vi "CRYNot.ch Resonance.vi"(8 "Y ref":dbl=1.0, 9 "Curve in":cluster{"x":dbl, "y":dbl, "z":dbl}[](array[cluster]) {"z" format="%.2f"; "y" format="%.2f"; "x" format="%.2f"}, 10 "Fraction down (1/sqrt(2))":dbl=0.2928932188134525 format="%.4f", 11 "Y data":dbl=1.0) -> (1 "Index":i32, 3 "Interval around max":cluster{"Freq":dbl, "Magn":dbl}[](array[cluster]) {"Magn" format="%.4f"; "Freq" format="%.2f"})   [LabVIEW 2013]
panel:
  in  "In L(f)":dbl
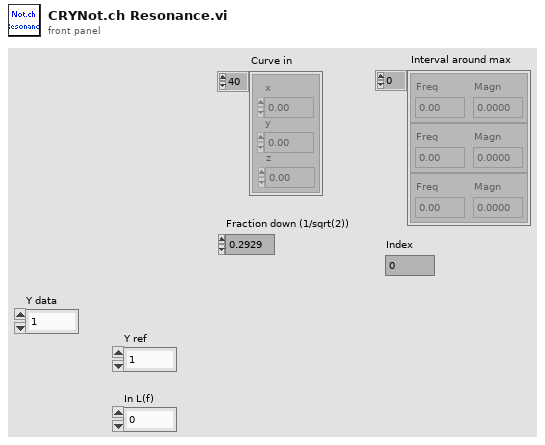
[diagram p1: front panel]
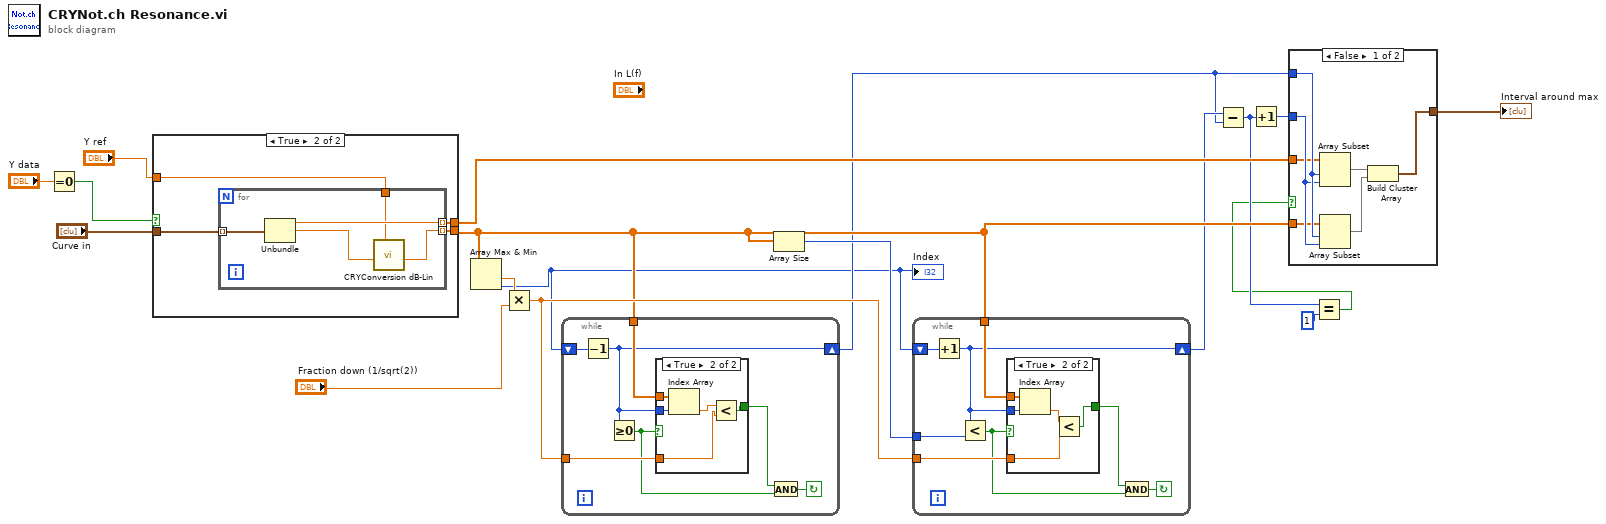
[diagram p0: block diagram]
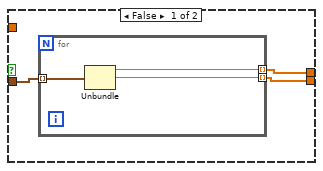
[diagram p2: hidden frame]
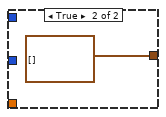
[diagram p3: hidden frame]
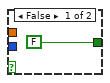
[diagram p4: hidden frame]
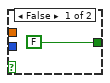
[diagram p5: hidden frame]
diagram:
  n1 = Equal To 0?(x="Y data") -> (x = 0?=w6:bool)
  n2 = case shown="True" w6 {
    tunnel: [w19 w28] -> w16
    tunnel: [w20 w27] -> w15
    tunnel: "Curve in" -> [w21 w26]
    tunnel: "Y ref" -> [_ w25]
    frame False {
      n3 = for {
        tunnel: w21 -> [w24] mode=indexing
        tunnel: [w22] -> w19 mode=indexing
        tunnel: [w23] -> w20 mode=indexing
        n4 = Unbundle(w24) -> ("x"=w23:dbl, "y"=w22:dbl)  [unwired: 1 out]
      }
    }
    frame True {
      n5 = for {
        tunnel: w26 -> [w33] mode=indexing
        tunnel: [w30] -> w28 mode=indexing
        tunnel: [w32] -> w27 mode=indexing
        tunnel: w25 -> [w29]
        n6 = Unbundle(w33) -> ("x"=w32:dbl, "y"=w31:dbl)  [unwired: 1 out]
        n7 = call "CRYConversion dB-Lin.vi"("dB ref."=w29, "Log In"=w31) -> ("Lin Out"=w30:dbl)  [unwired: 4 in, 3 out]
      }
    }
  }
  n8 = Array Max & Min(array=w16) -> (min value=w2:dbl, min index (indices)=w1:i32)  [unwired: 2 out]
  "Index" <- w1
  n9 = Multiply(x=w2, y="Fraction down (1/sqrt(2))") -> (x*y=w17:dbl)
  n10 = while {
    shift-right: [w35] -> w12
    shift-left: w1 -> [w40]
    tunnel: w17 -> [w38]
    tunnel: w16 -> [w39]
    stop <- w36 continue-if-true
    n11 = Decrement(x=w40) -> (x-1=w35:i32)
    n12 = Greater Or Equal To 0?(x=w35) -> (x >= 0?=w34:bool)
    n13 = case shown="True" w34 {
      tunnel: w39 -> [_ w46]
      tunnel: w35 -> [_ w45]
      tunnel: w38 -> [_ w43]
      tunnel: [FALSE w42] -> w37
      frame False {
      }
      frame True {
        n14 = Index Array(array=w46, index=w45) -> (element=w44:dbl)
        n15 = Less?(x=w44, y=w43) -> (x < y?=w42:bool)
      }
    }
    n16 = And(x=w37, y=w34) -> (x .and. y?=w36:bool)
  }
  n17 = Array Size(array=w16) -> (size(s)=w18:i32)
  n18 = while {
    shift-right: [w49] -> w13
    shift-left: w1 -> [w54]
    tunnel: w17 -> [w52]
    tunnel: w16 -> [w53]
    tunnel: w18 -> [w48]
    stop <- w50 continue-if-true
    n19 = Increment(x=w54) -> (x+1=w49:i32)
    n20 = Less?(x=w49, y=w48) -> (x < y?=w47:bool)
    n21 = case shown="True" w47 {
      tunnel: w53 -> [_ w60]
      tunnel: w49 -> [_ w59]
      tunnel: w52 -> [_ w58]
      tunnel: [FALSE w56] -> w51
      frame False {
      }
      frame True {
        n22 = Index Array(array=w60, index=w59) -> (element=w57:dbl)
        n23 = Less?(x=w57, y=w58) -> (x < y?=w56:bool)
      }
    }
    n24 = And(x=w51, y=w47) -> (x .and. y?=w50:bool)
  }
  n25 = Subtract(x=w13, y=w12) -> (x-y=w4:i32)
  n26 = Increment(x=w4) -> (x+1=w11:i32)
  n27 = Equal?(x=w4, y=1) -> (x = y?=w3:bool)
  n28 = case shown="False" w3 {
    tunnel: w12 -> [w67 _]
    tunnel: w16 -> [w64 _]
    tunnel: w15 -> [w65 _]
    tunnel: [w61 cluster{"Freq":dbl, "Magn":dbl}[] [] ("Interval around max")] -> w14
    tunnel: w11 -> [w66 _]
    frame False {
      n29 = Array Subset(array=w65, index=w67, length=w66) -> (w63:dbl[])
      n30 = Array Subset(array=w64, index=w67, length=w66) -> (w62:dbl[])
      n31 = Build Cluster Array(w63, w62) -> (w61:cluster{"x":dbl, "Lin Out":dbl}[])
    }
    frame True {
    }
  }
  "Interval around max" <- w14
